vi "FTW-Example-Actors-RT.vi"() -> ()   [LabVIEW 2013]
uses:
  Actor/src/Connector/FTW-ActorConnector.lvclass
  Actor/src/Ether/FTW-Ether.lvclass
panel:
  in  "Boolean":bool
  out "Instance Publisher Address":string
  out "Instance Inbox Address":string
  out "Initialized Response":string
  out "Timed out?":bool
  out "Ping Response":string
  in  "FTW Ether Configuration":string="{\n  \"ApplicationName\": \"Actor Example\",\n  \"ApplicationVersion\": \"0.1.0-1\",\n  \"LoggerAddress\": \"lvq://*\",\n  \"LoggerName\": \"ActorExample\",\n  \"LoggerDirectory\": \"/c/logs\",\n  \"LoggerDiskThrashDelay\": 200\n}"
  in  "Actor 1 Configuration":string="{\n  \"Identity\": \"FeatherweightActorExample\",\n  \"InboxAddress\": \"lvq://*\",\n  \"PublisherAddress\": \"lvn://*\",\n  \"LoggerAddress\": \"\",\n  \"DebugEnableInboxLogging\": false,\n  \"DebugEnableJobLogging\": false,\n  \"DebugShowPanel\": false\n}"
  out "error out":errorcluster
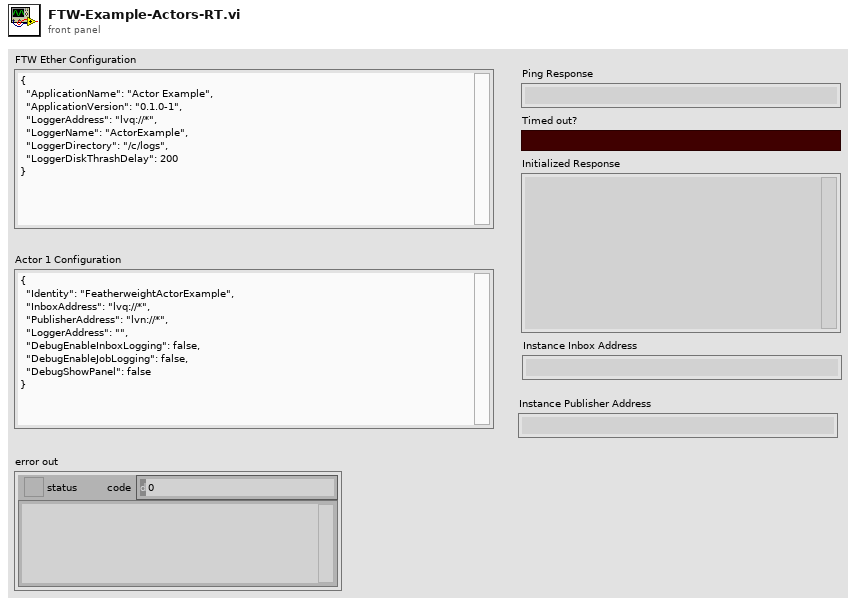
[diagram p1: front panel]
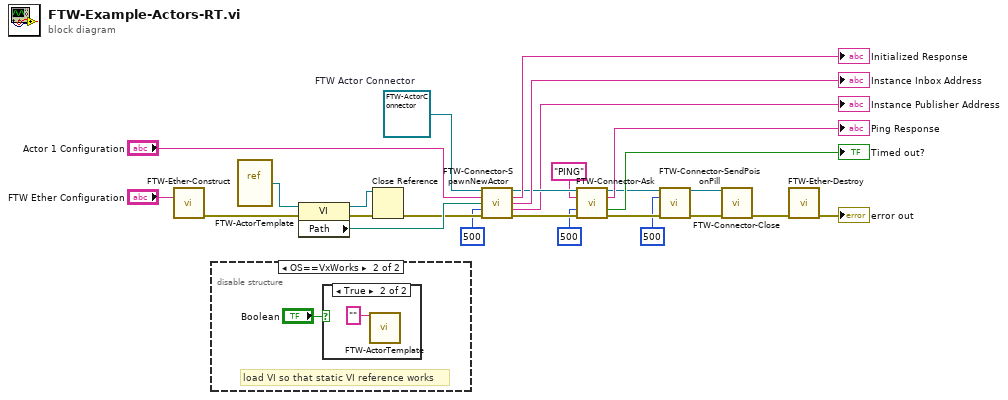
[diagram p0: block diagram]
diagram:
  w17 = refnum<class "FTW-ActorConnector.lvclass"> refnum  # FTW Actor Connector
  n1 = call "FTW-Ether-Construct.vi"("FTW Ether Configuration"="FTW Ether Configuration") -> ("error out"=w25:errorcluster)  [unwired: 14 in]
  n2 = disable-structure shown="OS==VxWorks" {
    frame condition #0 {
    }
    frame condition #1 (active) {
      # "load VI so that static VI reference works"
      n3 = case shown="True" "Boolean" {
        frame False {
        }
        frame True {
          n4 = call "FTW-ActorTemplate.vi"("FTW Actor Instance Configuration"="") -> ()  [unwired: 14 in, 1 out]
        }
      }
    }
  }
  n5 = vi-ref "FTW-ActorTemplate.vi"() -> (w16:refnum<vi>)
  n6 = property class="VI"(reference=w16, error in=w25) -> (reference out=w6:refnum<vi>, error out=w5:errorcluster, "Path"=w15:path)
  n7 = Close Reference(reference=w6, error in (no error)=w5) -> (error out=w4:errorcluster)
  n8 = call "FTW-Connector-SpawnNewActor.vi"("FTW Actor Connector Type"=w17, "Configuration"="Actor 1 Configuration", "Actor VI Filepath"=w15, "Timeout"=500, "error in"=w4) -> ("FTW Actor Connector"=w14:refnum<class "FTW-ActorConnector.lvclass">, "Initialized Response"=→"Initialized Response":string, "Instance Inbox Address"=→"Instance Inbox Address":string, "Instance Publisher Address"=→"Instance Publisher Address":string, "error out"=w13:errorcluster)  [unwired: 6 in]
  n9 = call "FTW-Connector-Ask.vi"("FTW Actor Connector"=w14, "Request Header"="PING", "Timeout"=500, "error in"=w13) -> ("FTW Actor Connector out"=w11:refnum<class "FTW-ActorConnector.lvclass">, "Response Header"=→"Ping Response":string, "Timed out?"=→"Timed out?":bool, "error out"=w10:errorcluster)  [unwired: 7 in, 1 out]
  n10 = call-dynamic "FTW-Connector-SendPoisonPill.vi"("FTW Actor Connector"=w11, "Timeout"=500, "error in"=w10) -> ("FTW Actor Connector out"=w9:refnum<class "FTW-ActorConnector.lvclass">, "error out"=w8:errorcluster)  [unwired: 8 in, 3 out]
  n11 = call-dynamic "FTW-Connector-Close.vi"("FTW Actor Connector"=w9, "error in"=w8) -> ("error out"=w21:errorcluster)  [unwired: 13 in]
  n12 = call "FTW-Ether-Destroy.vi"("error in"=w21) -> ("error out"=→"error out":errorcluster)  [unwired: 14 in]
